vi "MB Status Manager.vi"(0 "start in":bool, 1 "connect in":bool, 2 "write enable in":bool, 3 "Remote Param in":T1={"Remote IP Address"="192.168.254.254", "Remote Port"=502}, 4 "errors":u16, 5 "error in (no error)":errorcluster, 6 "Table":T2(ring), 7 "N":i32, 8 "Function":T3(ring)=enum."Read", 9 "Length":i32=1 min=1) -> (14 "start":bool, 15 "connect":bool[](array[boolean]), 16 "write enable":bool, 17 "Remote Param":T1={"Remote IP Address"="192.168.254.254", "Remote Port"=502}, 18 "Errors":u16[](array[numeric]), 19 "error out":errorcluster)   [LabVIEW 2019, in "NI_modbus_upd.lvlib"]
uses:
  NI_modbus_upd.lvlib
panel:
  # "VI Name: MB Registers Manager.vi\nPurpose: Read/Write Local Slave Registers."
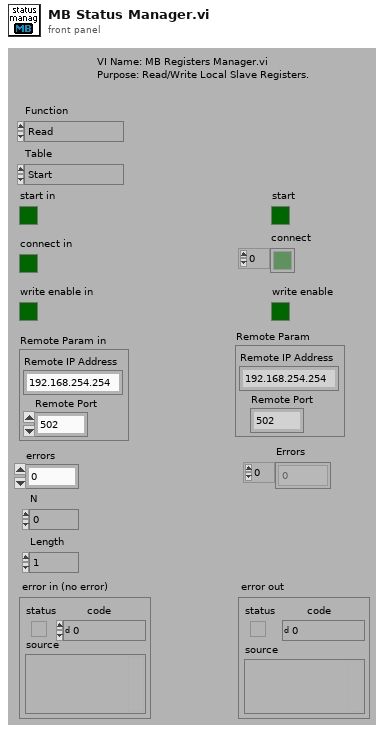
[diagram p1: front panel]
types:
  T1 = cluster{"Remote IP Address":string, "Remote Port":u16}
  T2 = enum16{"Start", "Connect", "Write enable", "IP address", "Errors"}
  T3 = enum16{"Init", "Read", "Read inputs", "Read outputs", "Write", "Write inputs"}
  T4 = cluster{"Remote IP Address":string, "Remote Port":u16}[]
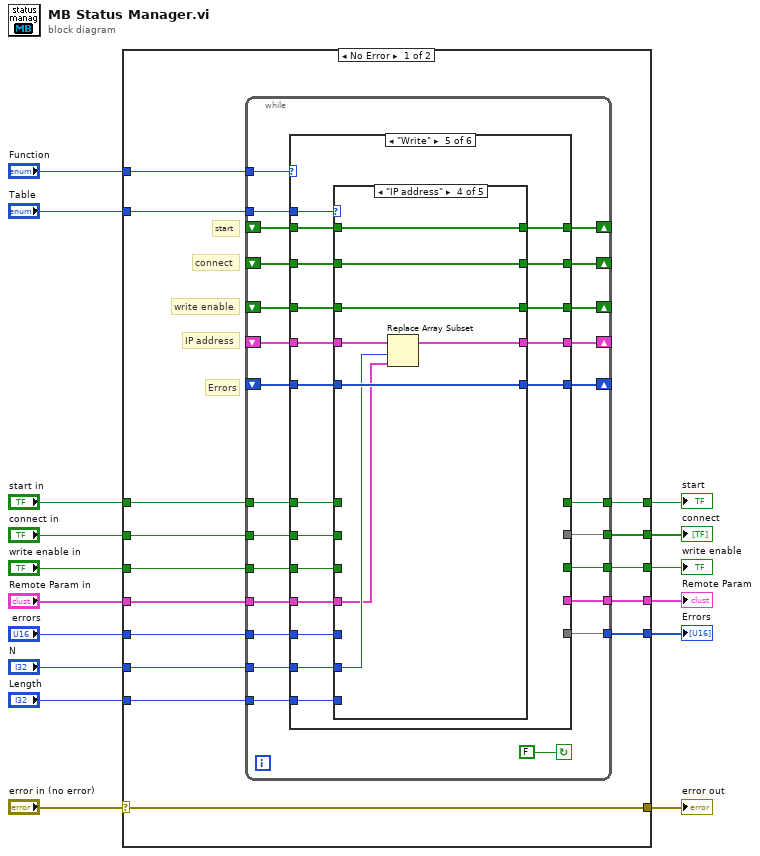
[diagram p0: block diagram]
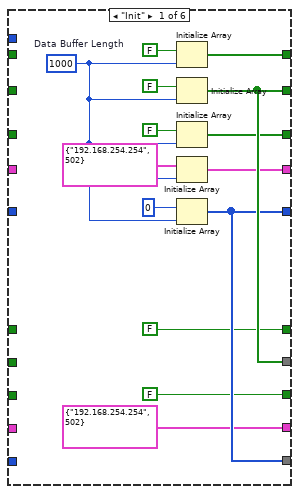
[diagram p2: hidden frame]
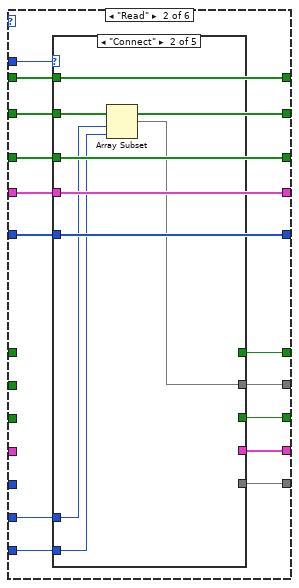
[diagram p3: hidden frame]
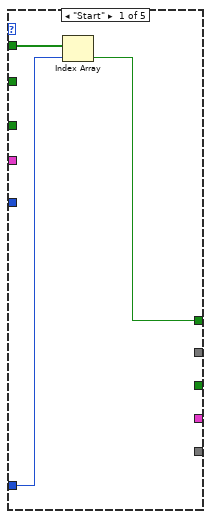
[diagram p4: hidden frame]
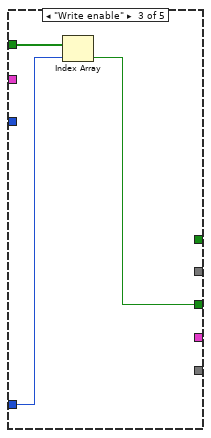
[diagram p5: hidden frame]
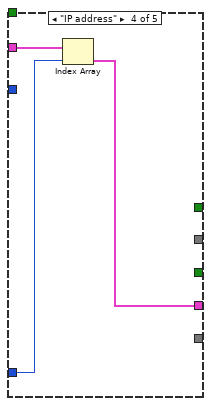
[diagram p6: hidden frame]
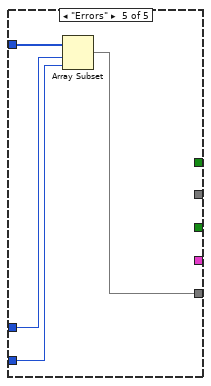
[diagram p7: hidden frame]
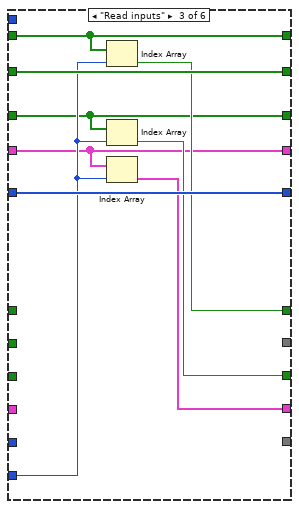
[diagram p8: hidden frame]
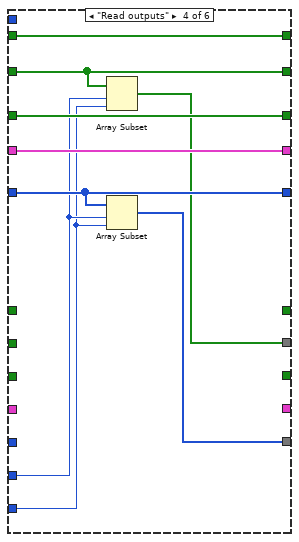
[diagram p9: hidden frame]
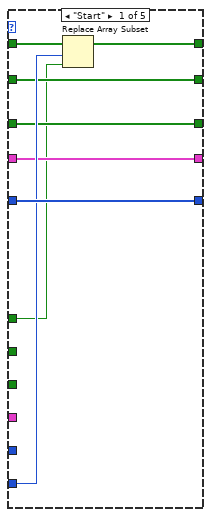
[diagram p10: hidden frame]
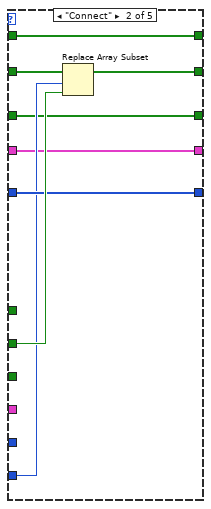
[diagram p11: hidden frame]
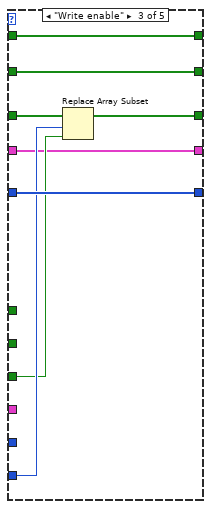
[diagram p12: hidden frame]
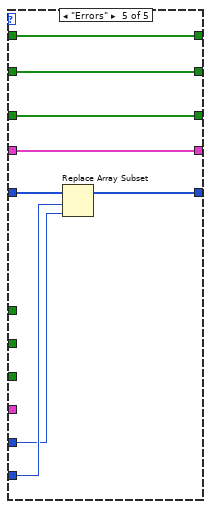
[diagram p13: hidden frame]
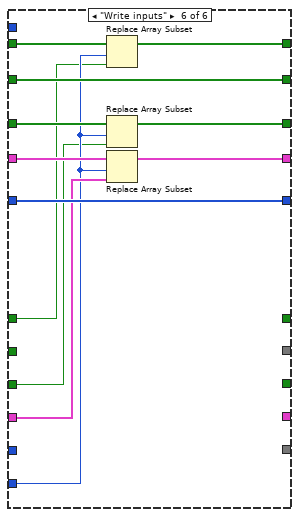
[diagram p14: hidden frame]
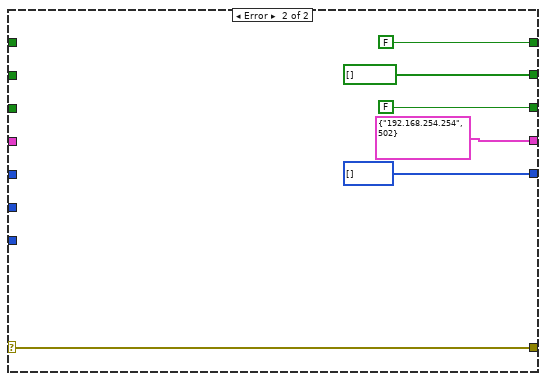
[diagram p15: hidden frame]
diagram:
  n1 = case shown="No Error" "error in (no error)" {
    selector: "error in (no error)" -> [w31 w194]
    tunnel: [w31 w194] -> w15
    tunnel: [w30 bool[] [] ("Bits In")] -> w14
    tunnel: [w29 u16[] []] -> w13
    tunnel: "Length" -> [w28 _]
    tunnel: "N" -> [w27 _]
    tunnel: "Function" -> [w26 _]
    tunnel: "Table" -> [w25 _]
    tunnel: "connect in" -> [w24 _]
    tunnel: "start in" -> [w23 _]
    tunnel: [w22 FALSE] -> w5
    tunnel: "errors" -> [w21 _]
    tunnel: [w20 FALSE] -> w4
    tunnel: "write enable in" -> [w19 _]
    tunnel: [w18 T1 {"Remote IP Address"="192.168.254.254", "Remote Port"=502} ("Remote Param")] -> w1
    tunnel: "Remote Param in" -> [w17 _]
    frame No Error {
      # "IP address"
      # "write enable"
      # "start"
      # "connect"
      # "Errors"
      n2 = while {
        tunnel: [w55] -> w30
        tunnel: [w54] -> w29
        tunnel: w28 -> [w53]
        tunnel: w27 -> [w52]
        tunnel: w26 -> [w51]
        shift-right: [w50] -> _
        shift-left: _ -> [w48]
        tunnel: w25 -> [w49]
        shift-right: [w47] -> _
        shift-left: _ -> [w46]
        tunnel: w24 -> [w45]
        shift-right: [w44] -> _
        shift-left: _ -> [w43]
        tunnel: w23 -> [w42]
        tunnel: [w41] -> w22
        tunnel: w21 -> [w40]
        shift-right: [w38] -> _
        shift-left: _ -> [w39]
        tunnel: [w37] -> w20
        tunnel: w19 -> [w36]
        shift-right: [w35] -> _
        shift-left: _ -> [w34]
        tunnel: [w33] -> w18
        tunnel: w17 -> [w32]
        stop <- FALSE continue-if-true
        n3 = case shown="\"Write\"" w51 {
          tunnel: w52 -> [_ w82 w105 w113 w135 w179]
          tunnel: [w67 w79 _ w110 _ _] -> w54
          tunnel: [w68 w80 _ w111 _ _] -> w55
          tunnel: w53 -> [_ w81 _ w112 w134 _]
          tunnel: [w67 w78 w109 w115 w129 w187] -> w50
          tunnel: w49 -> [_ w83 _ _ w136 _]
          tunnel: w48 -> [_ w78 w109 w115 w133 w187]
          tunnel: [w68 w77 w108 w114 w130 w188] -> w47
          tunnel: w46 -> [_ w77 w108 w114 w132 w188]
          tunnel: w45 -> [_ _ _ _ w131 _]
          tunnel: [w65 w75 w104 w118 w127 w182] -> w44
          tunnel: w43 -> [_ w75 w104 w118 w128 w183]
          tunnel: w42 -> [_ _ _ _ w126 w178]
          tunnel: [FALSE w76 w107 _ _ _] -> w41
          tunnel: w40 -> [_ _ _ _ w125 _]
          tunnel: [w64 w74 w103 w117 w124 w180] -> w38
          tunnel: w39 -> [_ w74 w103 w117 w123 w181]
          tunnel: [FALSE w73 w106 _ _ _] -> w37
          tunnel: w36 -> [_ _ _ _ w122 w177]
          tunnel: [w60 w72 w102 w116 w121 w186] -> w35
          tunnel: w34 -> [_ w72 w102 w116 w120 w185]
          tunnel: [T1 {"Remote IP Address"="192.168.254.254", "Remote Port"=502} ("Remote Param") w71 w101 _ _ _] -> w33
          tunnel: w32 -> [_ _ _ _ w119 w184]
          frame "Init" {
            w59 = 1000  # Data Buffer Length
            n4 = Initialize Array(FALSE, w59) -> (w65:bool[])
            n5 = Initialize Array(FALSE, w59) -> (w68:bool[])
            n6 = Initialize Array(FALSE, w59) -> (w64:bool[])
            n7 = Initialize Array(T1 {"Remote IP Address"="192.168.254.254", "Remote Port"=502} ("Remote Param"), w59) -> (w60:T4)
            n8 = Initialize Array(u16 0, w59) -> (w67:u16[])
          }
          frame "Read" {
            n9 = case shown="\"Connect\"" w83 {
              tunnel: w82 -> [w84 w88 w91 w95 w100]
              tunnel: w81 -> [_ w87 _ _ w97]
              tunnel: [_ w89 _ _ _] -> w80
              tunnel: [_ _ _ _ w98] -> w79
              tunnel: w78 -> [_ _ _ _ w99]
              tunnel: w77 -> [_ w90 _ _ _]
              tunnel: [w85 _ _ _ _] -> w76
              tunnel: w75 -> [w86 _ _ _ _]
              tunnel: w74 -> [_ _ w93 _ _]
              tunnel: [_ _ w92 _ _] -> w73
              tunnel: w72 -> [_ _ _ w96 _]
              tunnel: [_ _ _ w94 _] -> w71
              frame "Start" {
                n10 = Index Array(array=w86, index=w84) -> (element=w85:bool)
              }
              frame "Connect" {
                n11 = Array Subset(array=w90, index=w88, length=w87) -> (w89:bool[])
              }
              frame "Write enable" {
                n12 = Index Array(array=w93, index=w91) -> (element=w92:bool)
              }
              frame "IP address" {
                n13 = Index Array(array=w96, index=w95) -> (element=w94:T1)
              }
              frame "Errors" {
                n14 = Array Subset(array=w99, index=w100, length=w97) -> (w98:u16[])
              }
            }
          }
          frame "Read inputs" {
            n15 = Index Array(array=w104, index=w105) -> (element=w107:bool)
            n16 = Index Array(array=w103, index=w105) -> (element=w106:bool)
            n17 = Index Array(array=w102, index=w105) -> (element=w101:T1)
          }
          frame "Read outputs" {
            n18 = Array Subset(array=w114, index=w113, length=w112) -> (w111:bool[])
            n19 = Array Subset(array=w115, index=w113, length=w112) -> (w110:u16[])
          }
          frame "Write" {
            n20 = case shown="\"IP address\"" w136 {
              tunnel: w135 -> [w143 w148 w159 w167 w176]
              tunnel: w134 -> [_ _ _ _ _]
              tunnel: w133 -> [w144 w149 w160 w168 w175]
              tunnel: w132 -> [w140 w152 w155 w164 w174]
              tunnel: w131 -> [_ w151 _ _ _]
              tunnel: [w140 w150 w155 w164 w174] -> w130
              tunnel: [w144 w149 w160 w168 w173] -> w129
              tunnel: w128 -> [w142 w147 w158 w165 w172]
              tunnel: [w141 w147 w158 w165 w172] -> w127
              tunnel: w126 -> [w137 _ _ _ _]
              tunnel: w125 -> [_ _ _ _ w171]
              tunnel: [w139 w146 w156 w163 w170] -> w124
              tunnel: w123 -> [w139 w146 w157 w163 w170]
              tunnel: w122 -> [_ _ w154 _ _]
              tunnel: [w138 w145 w153 w161 w169] -> w121
              tunnel: w120 -> [w138 w145 w153 w162 w169]
              tunnel: w119 -> [_ _ _ w166 _]
              frame "Start" {
                n21 = Replace Array Subset(array=w142, new element=w137, index=w143) -> (w141:bool[])
              }
              frame "Connect" {
                n22 = Replace Array Subset(array=w152, new element=w151, index=w148) -> (w150:bool[])
              }
              frame "Write enable" {
                n23 = Replace Array Subset(array=w157, new element=w154, index=w159) -> (w156:bool[])
              }
              frame "IP address" {
                n24 = Replace Array Subset(array=w162, new element=w166, index=w167) -> (w161:T4)
              }
              frame "Errors" {
                n25 = Replace Array Subset(array=w175, new element=w171, index=w176) -> (w173:u16[])
              }
            }
          }
          frame "Write inputs" {
            n26 = Replace Array Subset(array=w183, new element=w178, index=w179) -> (w182:bool[])
            n27 = Replace Array Subset(array=w181, new element=w177, index=w179) -> (w180:bool[])
            n28 = Replace Array Subset(array=w185, new element=w184, index=w179) -> (w186:T4)
          }
        }
      }
    }
    frame Error {
    }
  }
  "error out" <- w15
  "connect" <- w14
  "Errors" <- w13
  "start" <- w5
  "write enable" <- w4
  "Remote Param" <- w1
